vi "SEK2020v1SubVISeguidorLinha.vi"(8 "Parâmetros":T1={"Azul Max EV3 Cor"=17, "Azul Min EV3 Cor"=0, "Verde Max EV3 Cor"=6, "Verde Min EV3 Cor"=0, "Vermelho Max Ev3 Cor"=0, "Vermelho Min EV3 Cor"=0, "Chão EV3 Cor"=0.0, "Branco Max EV3 Cor"=0.0, "Branco Min EV3 Cor"=0.0, "Preto Max EV3 Cor"=0.0, "Preto Min EV3 Cor"=0.0, "Distância Tubulação"=0.0, "Distância Frontal"=0.0, "Amarelo Max EV3 Cor"=0.0, "Amarelo Min EV3 Cor"=0.0, "Distância Lateral"=0.0, "90°"=0.0, "180°"=0.0, "Seguidor de Linha"=0.0}, 10 "NXT/EV3":T2) -> (2 "NXT/EV3 3":T2)   [LabVIEW 2016]
uses:
  <vilib>/NXT/Subs/LVHSConnector.ctl
  <vilib>/NXT/LegoClasses/BrickReference/BrickReference.lvclass
  <vilib>/NXT/Block Support/NXT_InputPort.ctl
  <vilib>/NXT/Block Support/NXT_OutputPort.ctl
  <vilib>/NXT/Dual Mode Library/Sensors/EV3_Color_Reflect.vi
  <vilib>/NXT/NXTIO Xnodes/NXTIONodeSubVIs/NXTMoveMotors.vi
  <vilib>/NXT/NXTIO Xnodes/NXTIONodeSubVIs/NXTStopMotors.vi
  <vilib>/NXT/NXTIO Xnodes/AddressXNode/NXTIOAddress.xnode
  <vilib>/NXT/NXTIO Xnodes/NXTIOXNode/NXTIO.xnode
panel:
  in  "constante p":dbl format="%#_13g"
  # "Sensor EV3 Cor"
  # "Sensor Ultrassônico"
  # "Sensor Giroscópio"
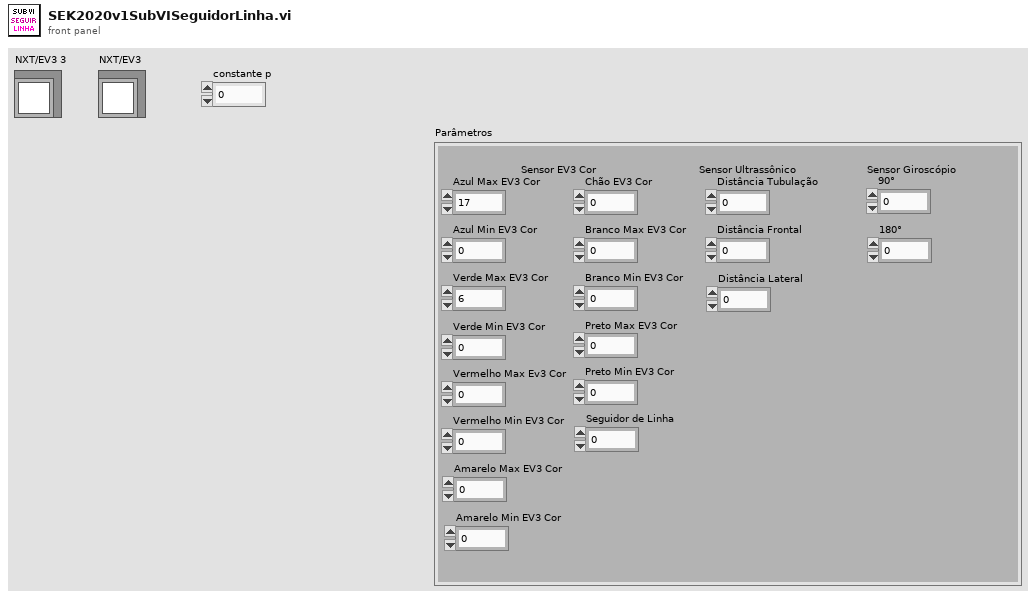
[diagram p1: front panel]
types:
  T1 = cluster{"Azul Max EV3 Cor":i32, "Azul Min EV3 Cor":i32, "Verde Max EV3 Cor":i32, "Verde Min EV3 Cor":i32, "Vermelho Max Ev3 Cor":i32, "Vermelho Min EV3 Cor":i32, "Chão EV3 Cor":sgl, "Branco Max EV3 Cor":sgl, "Branco Min EV3 Cor":sgl, "Preto Max EV3 Cor":sgl, "Preto Min EV3 Cor":sgl, "Distância Tubulação":sgl, "Distância Frontal":sgl, "Amarelo Max EV3 Cor":dbl, "Amarelo Min EV3 Cor":dbl, "Distância Lateral":sgl, "90°":sgl, "180°":sgl, "Seguidor de Linha":dbl}
  T2 = typedef "LVHSConnector.ctl" = refnum<class "BrickReference.lvclass">
  T3 = typedef "NXT_OutputPort.ctl" = u8
  T4 = typedef "NXT_InputPort.ctl" = u32
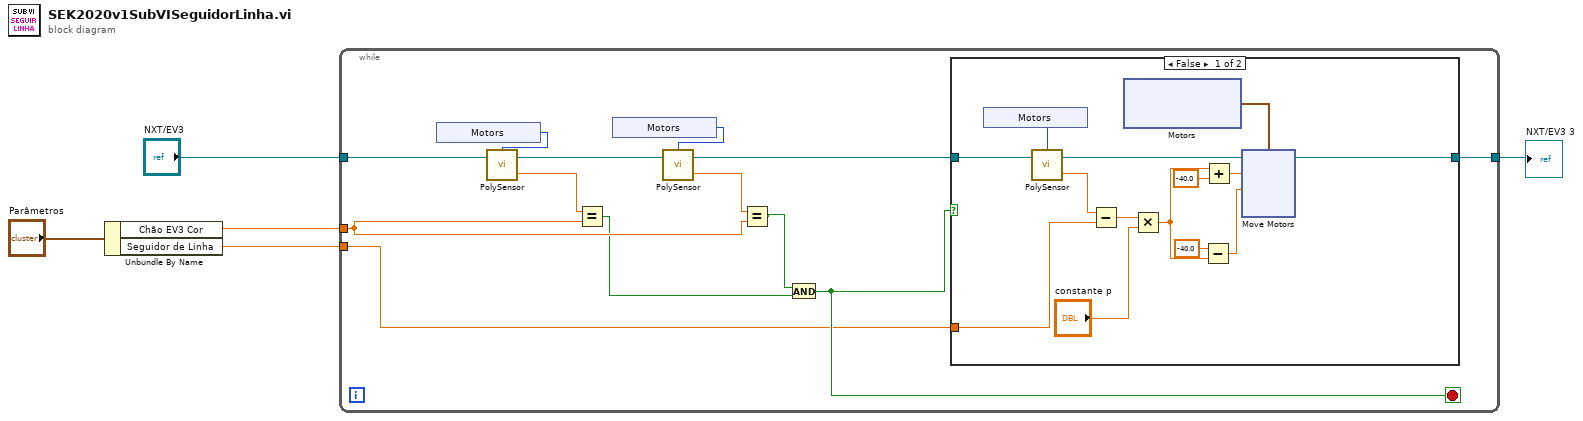
[diagram p0: block diagram]
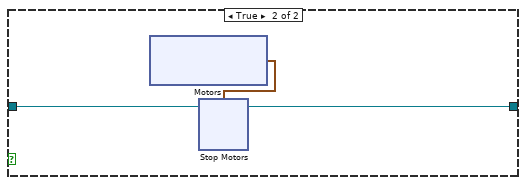
[diagram p2: hidden frame]
diagram:
  n1 = Unbundle By Name("Parâmetros") -> ("Chão EV3 Cor"=w2:sgl, "Seguidor de Linha"=w1:dbl)
  n2 = while {
    tunnel: "NXT/EV3" -> [w15]
    tunnel: [w14] -> w4
    tunnel: w2 -> [w7]
    tunnel: w1 -> [w8]
    stop <- w13 stop-if-true
    n3 = xnode "Motors"() -> ("Sensor"=w18:T4)
    n4 = call-poly <vilib>:"PolySensor.vi"("NXT/EV3"=w15, "Port (Port 1)"=w18) -> ("Scaled Value"=w9:sgl, "NXT/EV3"=w16:T2)  [unwired: 1 in]
    n5 = Equal?(x=w9, y=w7) -> (x = y?=w6:bool)
    n6 = xnode "Motors"() -> ("Sensor"=w17:T4)
    n7 = call-poly <vilib>:"PolySensor.vi"("NXT/EV3"=w16, "Port (Port 1)"=w17) -> ("Scaled Value"=w10:sgl, "NXT/EV3"=w12:T2)  [unwired: 1 in]
    n8 = Equal?(x=w10, y=w7) -> (x = y?=w11:bool)
    n9 = And(x=w11, y=w6) -> (x .and. y?=w13:bool)
    n10 = case shown="False" w13 {
      tunnel: [w20 w44] -> w14
      tunnel: w12 -> [w22 w45]
      tunnel: w8 -> [w19 _]
      frame False {
        n11 = xnode "Motors"() -> ("Sensor"=w25:T4)
        n12 = call-poly <vilib>:"PolySensor.vi"("NXT/EV3"=w22, "Port (Port 1)"=w25) -> ("Scaled Value"=w32:sgl, "NXT/EV3"=w26:T2)  [unwired: 1 in]
        n13 = Subtract(x=w32, y=w19) -> (x-y=w31:dbl)
        n14 = xnode "Motors"() -> ("Motor"=w21:cluster{"Port":T3, "Port":T3})
        n15 = Multiply(x=w31, y="constante p") -> (x*y=w23:dbl)
        n16 = Subtract(x=-40.0 ("y"), y=w23) -> (x-y=w27:dbl)
        n17 = Add(x=w23, y=-40.0) -> (x+y=w28:dbl)
        n18 = xnode "Move Motors"("Power/Speed 2"=w27, "Power/Speed 1"=w28, "Motors"=w21, "NXT/EV3"=w26) -> ("NXT/EV3"=w20:T2)
      }
      frame True {
        n19 = xnode "Motors"() -> ("Motor"=w43:cluster{"Port":T3, "Port":T3})
        n20 = xnode "Stop Motors"("Motors"=w43, "NXT/EV3"=w45) -> ("NXT/EV3"=w44:T2)
      }
    }
  }
  "NXT/EV3 3" <- w4
